vi "Data_get_joe.vi"() -> ()   [LabVIEW 2011]
uses:
  <vilib>/Analysis/2dsp.llb/Real FFT.vi
  <vilib>/Analysis/NI_AALPro.lvlib
panel:
  out "f cur. (GHz)":i32
  in  "TDS VISA Port":refnum<visa-resource-name>="GPIB0::1::INSTR"
  in  "Chirp up to (GHz)":dbl
  in  "PauseB":bool caption="Pause"
  in  "Substr":bool
  out "tdsavges#":i32 caption="tds averaged:"
  in  "Auto":bool caption="Autosave"
  in  "FFT every#":u32=1 min=1 max=1000 step=1
  in  "#steps":u32=1 min=1 step=1
  in  "f step (MHz)":dbl=0.0003 min=0.00025 max=67.0 step=1e-06 format="%#.12f"
  in  "time/point":T1(ring)
  in  "time/div":T2(ring)
  out "Current sweep":u32=1 min=1 max=1000 step=1
  in  "Ext":string="ccd"
  in  "Name":string="trace"
  in  "Folder":path
  in  "#Sweeps":u32=1 min=1 max=1000 step=1
  in  "Ampl. (dBm)":dbl min=-135.0 max=30.0 step=0.5 format="%#_8g"
  in  "f start (MHz)":dbl=0.0003 min=0.00025 max=67.0 step=1e-06 format="%#.12f"
  in  "Start":bool
  in  "Quit":bool
  in  "E8257D VISA Port":refnum<visa-resource-name>="GPIB0::1::INSTR"
  out "read time (ms)":u32
  out "#points":u32
  out "Busy":bool
  in  "Repetition rate (Hz)":ext=2.5
  in  "Chirp start (MHz)":ext=2.5
  in  "Filter up to (MHz)":ext=2.5
  in  "Amount of averagings":u32=10 min=1 step=1
  out "Data":dbl[](array[numeric])
  out "Frequency Domain Signal":cluster{ext[], dbl[]}(graph)
  out "FFT (Im)":dbl[](array[numeric])
  out "FFT (Re)":dbl[](array[numeric])
  out "Final array":ext[][](array[numeric])
  out "size(s)":i32
  out "Oscilloscope Data":dbl[](array[numeric])
  in  "Channel Number":u16=1
  out "Oscilloscope graph":dbl[](graph)
  in  "Stop":bool
  # "Oscilloscope TDS6124C"
  # "File Storage"
  # "PSG E8257D"
  # "Control"
  # "Spectrum data"
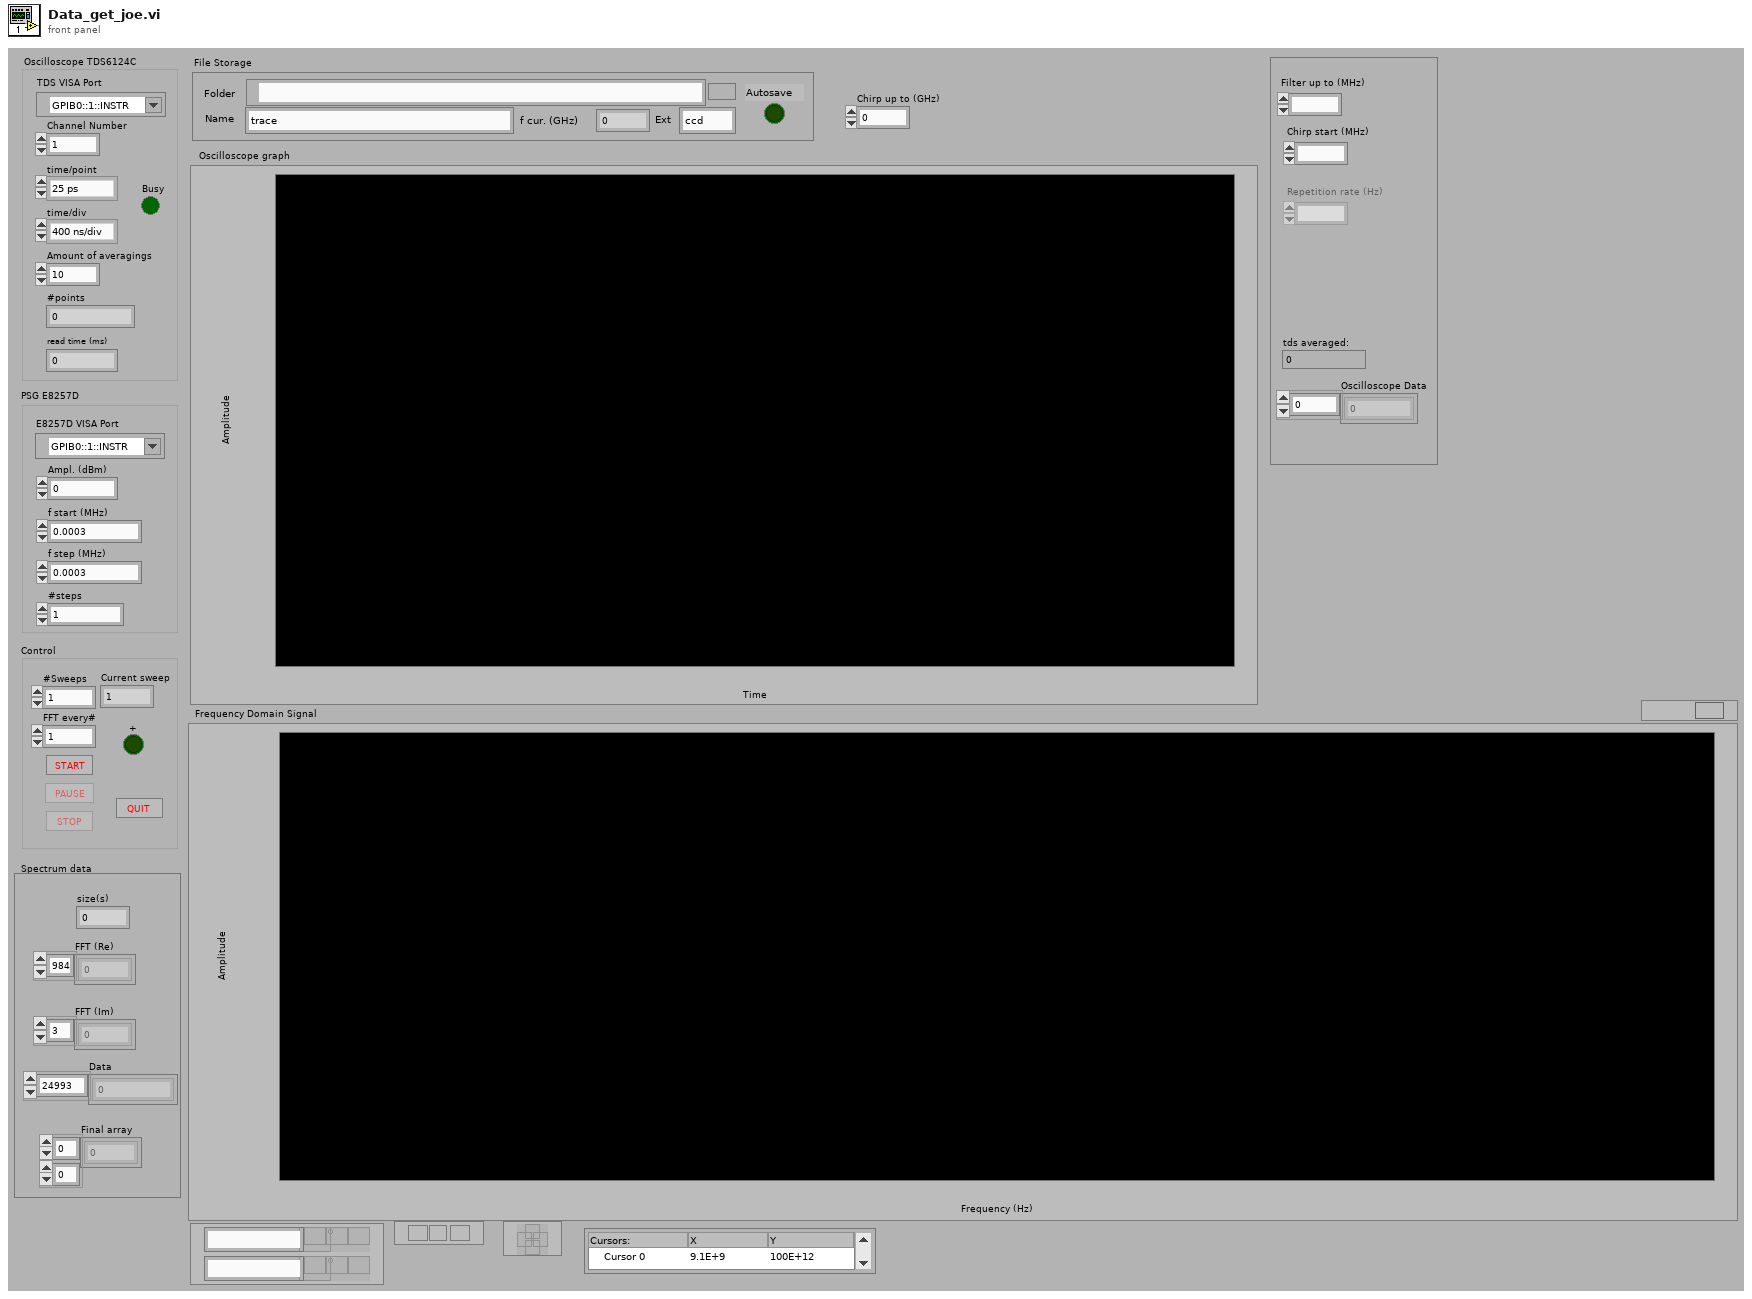
[diagram p1: front panel]
types:
  T1 = enum16{"25 ps", "50 ps", "100 ps", "200 ps", "400 ps", "800 ps", "2 ns"}
  T2 = enum16{"400 ns/div", "1 us/div", "2 us/div", "4 us/div", "10 us/div", "20 us/div"}
  T3 = enum8{"Enabled", "Disabled", "Disabled and Grayed Out"}
  T4 = enum16{"open", "replace", "create", "open or create", "replace or create", "replace or create with confirmation"}
  T5 = cluster{"Folder":path, "Name":string, "Ext":string}
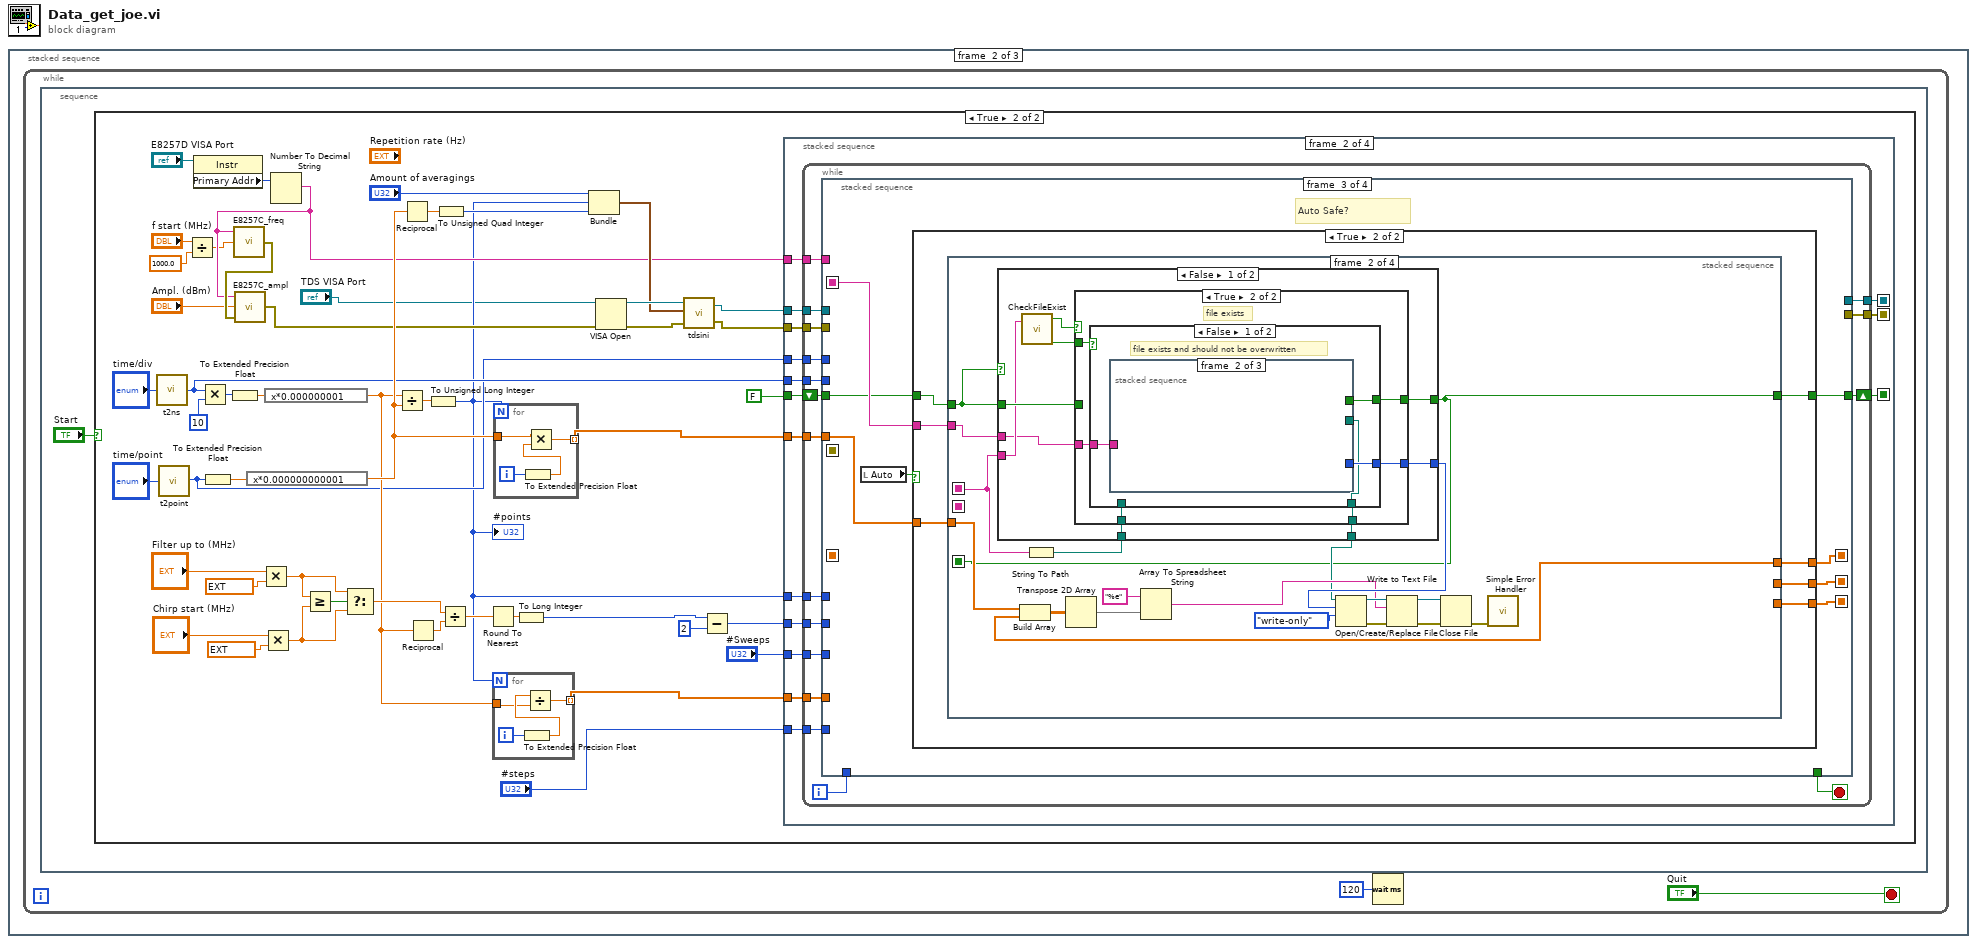
[diagram p0: block diagram]
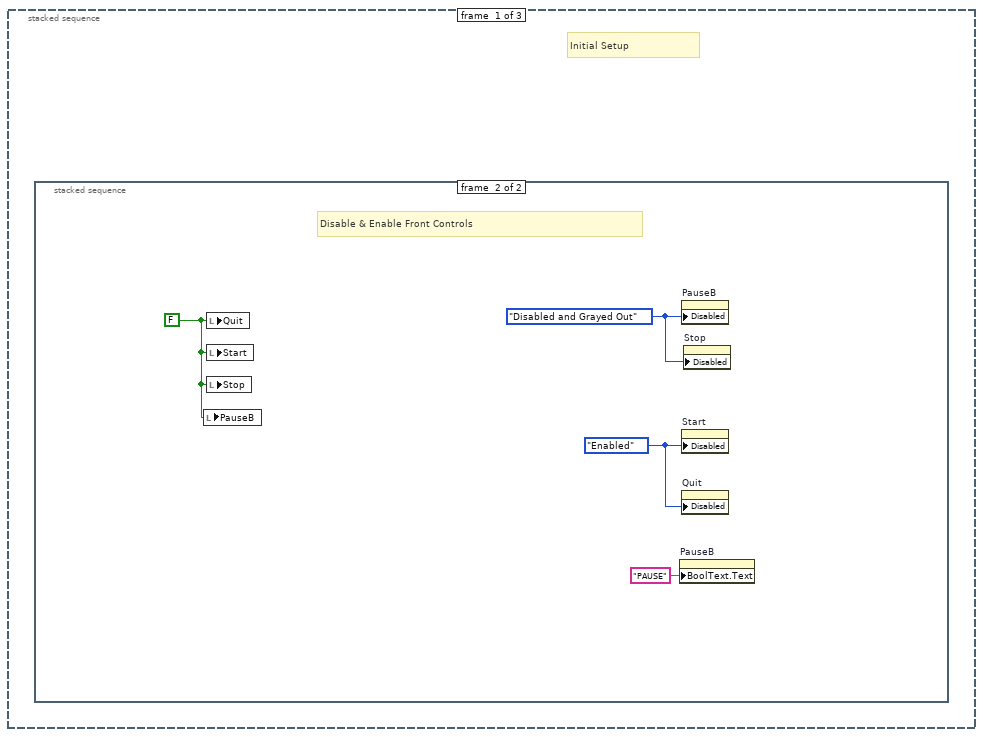
[diagram p2: hidden frame]
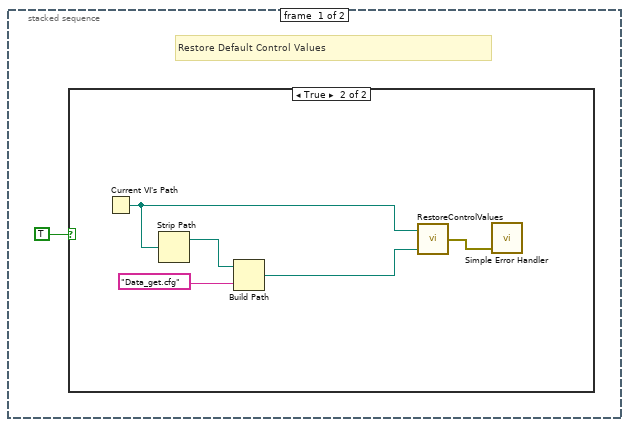
[diagram p3: hidden frame]
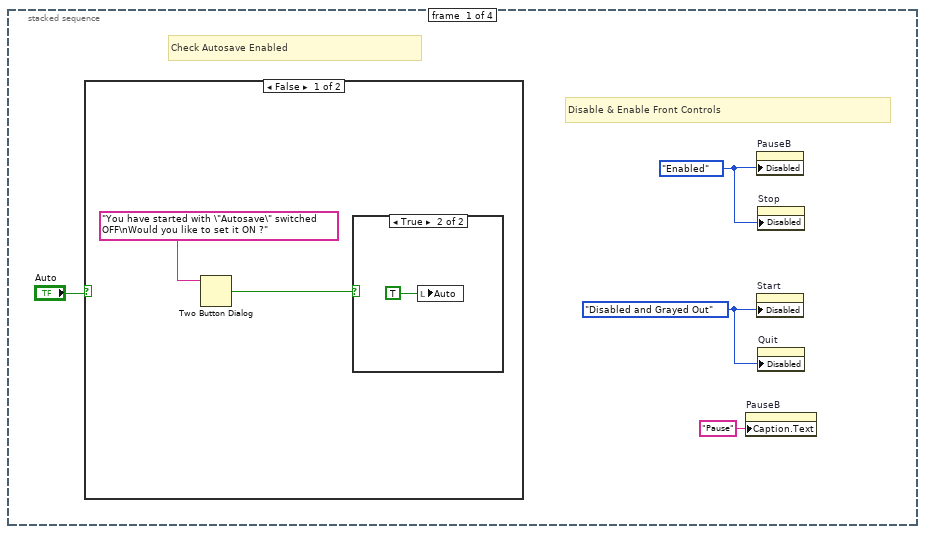
[diagram p6: hidden frame]
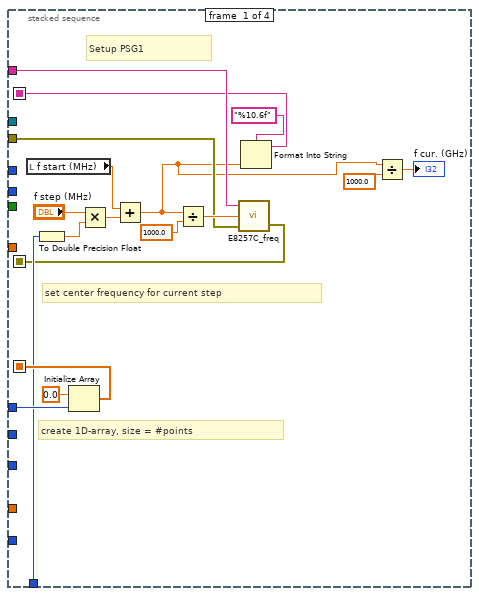
[diagram p9: hidden frame]
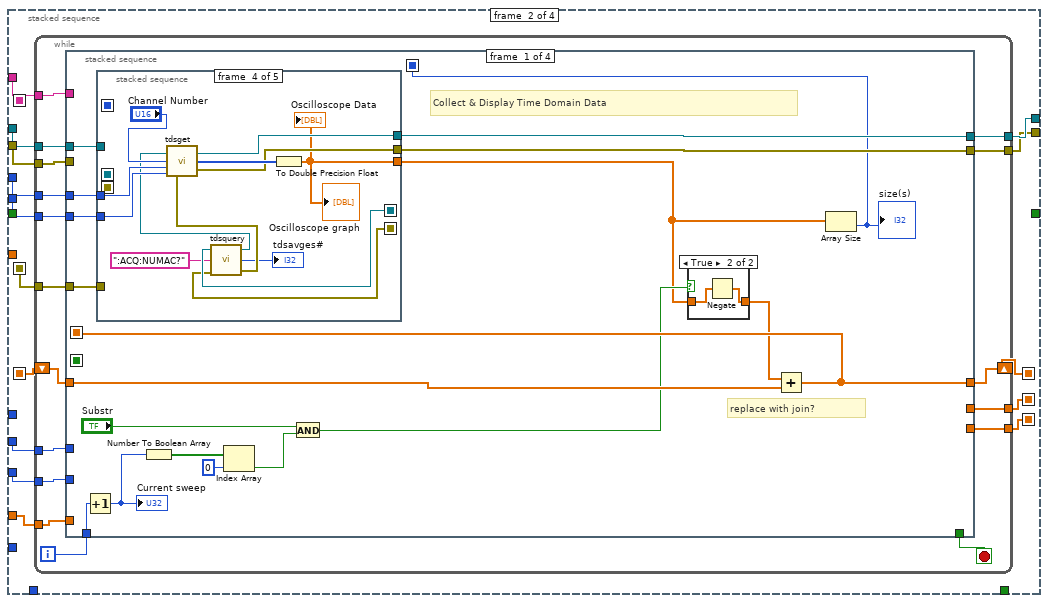
[diagram p10: hidden frame]
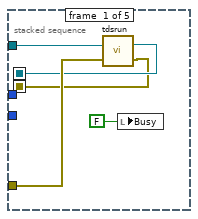
[diagram p12: hidden frame]
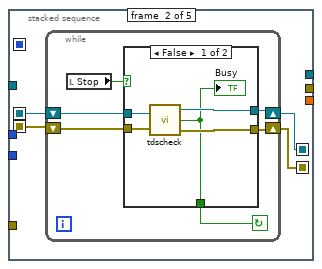
[diagram p13: hidden frame]
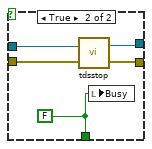
[diagram p14: hidden frame]
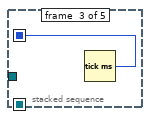
[diagram p15: hidden frame]
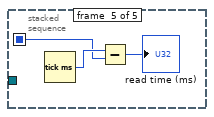
[diagram p16: hidden frame]
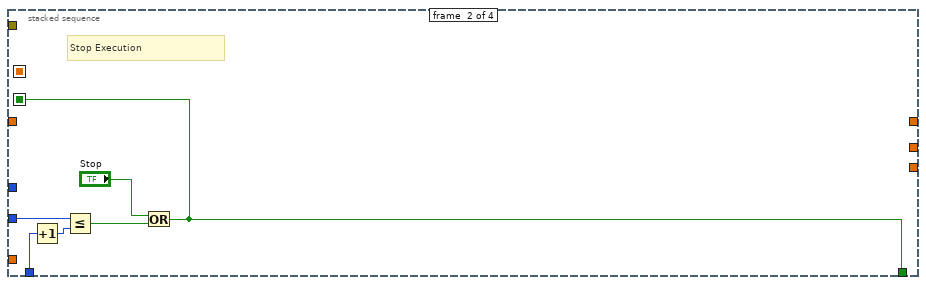
[diagram p17: hidden frame]
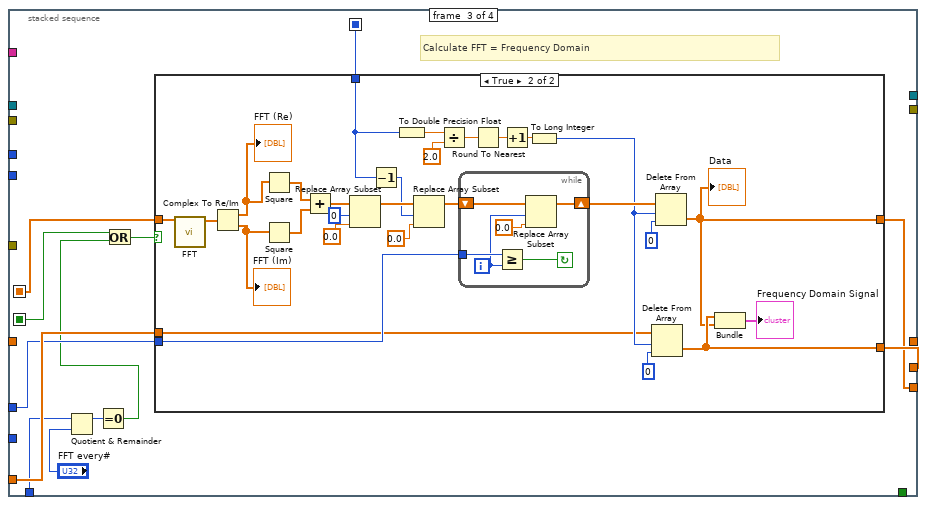
[diagram p18: hidden frame]
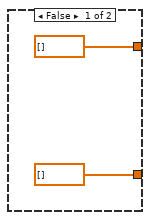
[diagram p19: hidden frame]
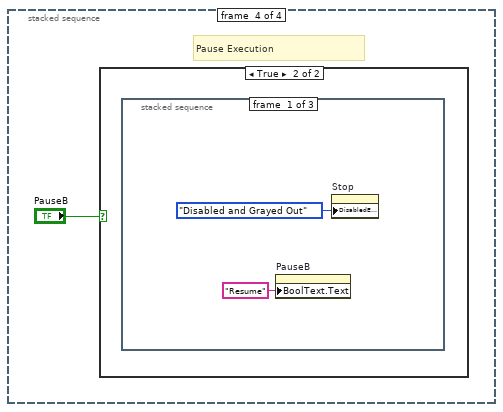
[diagram p20: hidden frame]
diagram:
  n1 = stacked-sequence {
    frame #0 {
      # "Initial Setup"
      n2 = stacked-sequence {
        frame #0 {
          # "Restore Default Control Values"
          n3 = case shown="True" TRUE {
            frame False {
            }
            frame True {
              n4 = Current VI's Path() -> (path=w2:path)
              n5 = Strip Path(path=w2) -> (stripped path=w3:path)  [unwired: 1 out]
              n6 = Build Path(base path=w3, name or relative path="Data_get.cfg") -> (appended path=w5:path)
              n7 = call "RestoreControlValues.vi"("file path"=w5, "vi path"=w2) -> ("error out"=w4:errorcluster)
              n8 = call <vilib>:"Simple Error Handler.vi"("error in (no error)"=w4) -> ()  [unwired: 4 in, 5 out]
            }
          }
        }
        frame #1 {
          w9 = T3."Disabled and Grayed Out" ("Disabled")
          w7 = T3."Enabled" ("Disabled")
          w10 = FALSE ("Quit")
          # "Disable & Enable Front Controls"
          n9 = local write "PauseB"(w10) -> ()
          n10 = local write "Quit"(w10) -> ()
          n11 = local write "Start"(w10) -> ()
          n12 = local write "Stop"(w10) -> ()
          n13 = property on="PauseB" class="Bool (strict)"("BoolText.Text"="PAUSE" ("Boolean Text.Text")) -> ()  [unwired: 2 in, 2 out]
          n14 = property on="PauseB" class="Bool (strict)"("Disabled"=w9) -> ()  [unwired: 2 in, 2 out]
          n15 = property on="Start" class="Bool (strict)"("Disabled"=w7) -> ()  [unwired: 2 in, 2 out]
          n16 = property on="Quit" class="Bool (strict)"("Disabled"=w7) -> ()  [unwired: 2 in, 2 out]
          n17 = property on="Stop" class="Bool (strict)"("Disabled"=w9) -> ()  [unwired: 2 in, 2 out]
        }
      }
    }
    frame #1 {
      n18 = while {
        stop <- "Quit" stop-if-true
        n19 = stacked-sequence {
          frame #0 {
            n20 = case shown="True" "Start" {
              frame False {
              }
              frame True {
                n21 = call "t2ns.vi"("t/div"="time/div") -> ("ns/div"=w25:u32)
                n22 = call "t2point.vi"("t/point"="time/point") -> ("ps/point"=w23:u32)
                n23 = Divide(x="f start (MHz)", y=1000.0) -> (x/y=w28:dbl)
                n24 = property class="Instr"(reference="E8257D VISA Port") -> ("Primary Addr"=w34:u16)  [unwired: 1 in, 2 out]
                n25 = Multiply(x=w25, y=u32 10) -> (x*y=w57:u32)
                n26 = To Extended Precision Float(1:w23) -> (0:w54:ext)
                n27 = To Extended Precision Float(1:w57) -> (0:w55:ext)
                n28 = expression code="x*0.000000000001"(w54) -> (w40:ext)
                n29 = Multiply(x="Filter up to (MHz)", y=ext 1000000.0) -> (x*y=w46:ext)
                n30 = Multiply(x="Chirp start (MHz)", y=ext 1000000.0) -> (x*y=w43:ext)
                n31 = expression code="x*0.000000001"(w55) -> (w36:ext)
                n32 = Number To Decimal String(number=w34) -> (decimal integer string=w31:string)  [unwired: 1 in]
                n33 = call "E8257C_freq.vi"("Frequency GHz"=w28, "GPIB address"=w31) -> ("error out"=w32:errorcluster)  [unwired: 1 in]
                n34 = call "E8257C_ampl.vi"("error in"=w32, "Amplitude dBm"="Ampl. (dBm)", "GPIB address"=w31) -> ("error out"=w30:errorcluster)
                n35 = Greater Or Equal?(x=w46, y=w43) -> (x >= y?=w53:bool)
                n36 = Select(t=w46, s=w53, f=w43) -> (s? t:f=w51:ext)
                n37 = Divide(x=w36, y=w40) -> (x/y=w56:ext)
                n38 = Reciprocal(x=w40) -> (1/x=w38:ext)
                n39 = Reciprocal(x=w36) -> (1/x=w52:ext)
                n40 = To Unsigned Long Integer(number=w56) -> (unsigned 32bit integer=w21:u32)
                "#points" <- w21
                n41 = To Unsigned Quad Integer(1:w38) -> (0:w39:u64)
                n42 = Divide(x=w51, y=w52) -> (x/y=w50:ext)
                n43 = Round To Nearest(number=w50) -> (nearest integer value=w49:ext)
                n44 = for {
                  N: w21 -> [_]
                  tunnel: w36 -> [w468]
                  tunnel: [w470] -> w37 mode=indexing
                  i -> [w471]
                  n45 = To Extended Precision Float(1:w471) -> (0:w469:ext)
                  n46 = Divide(x=w469, y=w468) -> (x/y=w470:ext)
                }
                n47 = for {
                  N: w21 -> [_]
                  tunnel: w40 -> [w473]
                  tunnel: [w472] -> w26 mode=indexing
                  i -> [w475]
                  n48 = To Extended Precision Float(1:w475) -> (0:w474:ext)
                  n49 = Multiply(x=w473, y=w474) -> (x*y=w472:ext)
                }
                n50 = To Long Integer(number=w49) -> (32bit integer=w18:i32)
                n51 = Bundle("Amount of averagings"="Amount of averagings", w21, w39) -> (w41:cluster{"Amount of averagings ":u32, u32, u64})  [unwired: 1 in]
                n52 = VISA Open(error in (no error)=w30, VISA resource name="TDS VISA Port") -> (VISA resource name=w59:refnum<visa-resource-name>, error out=w60:errorcluster)  [unwired: 3 in]
                n53 = call "tdsini.vi"("Error In (No Error)"=w60, "Acq_par"=w41, "VISA Port In"=w59) -> ("Error Out"=w61:errorcluster, "VISA Port Out"=w62:refnum<visa-resource-name>)
                n54 = Subtract(x=w18, y=2) -> (x-y=w16:i32)
                n55 = stacked-sequence {
                  seq-local: [_ w76 _ _] -> [_ _ w429 _]
                  seq-local: [_ w75 _ _] -> [_ _ w428 _]
                  seq-local: [_ w70 _ _] -> [_ _ _ w430]
                  tunnel: w62 -> [_ w84 _ _]
                  tunnel: w61 -> [_ w83 _ _]
                  tunnel: w23 -> [_ w82 _ _]
                  tunnel: w25 -> [_ w81 _ _]
                  tunnel: w16 -> [_ w80 _ _]
                  tunnel: w37 -> [_ w79 _ _]
                  tunnel: w31 -> [_ w78 w426 _]
                  tunnel: "#Sweeps" -> [_ w77 _ _]
                  tunnel: w26 -> [_ w72 _ _]
                  tunnel: w21 -> [_ w74 _ _]
                  tunnel: "#steps" -> [_ w73 _ _]
                  tunnel: FALSE -> [_ w71 _ _]
                  frame #0 {
                    w64 = T3."Enabled" ("Disabled")
                    w63 = T3."Disabled and Grayed Out" ("Disabled")
                    # "Check Autosave Enabled"
                    # "Disable & Enable Front Controls"
                    n56 = case shown="False" "Auto" {
                      frame False {
                        n57 = Two Button Dialog(message="You have started with \"Autosave\" switched OFF\nWould you like to set it ON ?") -> (T button?=w67:bool)  [unwired: 2 in]
                        n58 = case shown="True" w67 {
                          frame False {
                          }
                          frame True {
                            n59 = local write "Auto"(TRUE) -> ()
                          }
                        }
                      }
                      frame True {
                      }
                    }
                    n60 = property on="PauseB" class="Bool (strict)"("Caption.Text"="Pause") -> ()  [unwired: 2 in, 2 out]
                    n61 = property on="PauseB" class="Bool (strict)"("Disabled"=w64) -> ()  [unwired: 2 in, 2 out]
                    n62 = property on="Start" class="Bool (strict)"("Disabled"=w63) -> ()  [unwired: 2 in, 2 out]
                    n63 = property on="Stop" class="Bool (strict)"("Disabled"=w64) -> ()  [unwired: 2 in, 2 out]
                    n64 = property on="Quit" class="Bool (strict)"("Disabled"=w63) -> ()  [unwired: 2 in, 2 out]
                  }
                  frame #1 {
                    n65 = while {
                      tunnel: w84 -> [w101]
                      tunnel: w83 -> [w100]
                      tunnel: w82 -> [w99]
                      tunnel: w81 -> [w98]
                      tunnel: w80 -> [w97]
                      tunnel: w79 -> [w96]
                      tunnel: w78 -> [w95]
                      tunnel: w77 -> [w94]
                      tunnel: [w93] -> w76
                      tunnel: [w92] -> w75
                      tunnel: w74 -> [w91]
                      tunnel: w73 -> [w89]
                      tunnel: w72 -> [w87]
                      shift-right: [w85] -> w70
                      shift-left: w71 -> [w86]
                      i -> [w90]
                      stop <- w88 stop-if-true
                      n66 = stacked-sequence {
                        seq-local: [w118 _ _ _] -> [_ w124 _ _]
                        seq-local: [w107 _ _ _] -> [_ w123 _ _]
                        seq-local: [_ w122 _ _] -> [_ _ w282 _]
                        seq-local: [_ w121 _ _] -> [_ _ w281 _]
                        seq-local: [_ w120 _ _] -> [_ _ w280 _]
                        seq-local: [w105 _ _ _] -> [_ _ w279 _]
                        tunnel: w101 -> [_ w134 _ _]
                        tunnel: w100 -> [w108 w133 _ _]
                        tunnel: w99 -> [_ w132 _ _]
                        tunnel: w98 -> [_ w131 _ _]
                        tunnel: w97 -> [_ w130 _ _]
                        tunnel: w96 -> [_ w129 _ _]
                        tunnel: w95 -> [w109 w128 _ _]
                        tunnel: w94 -> [_ w127 _ _]
                        tunnel: [_ w126 _ _] -> w93
                        tunnel: [_ w125 _ _] -> w92
                        tunnel: w91 -> [w117 _ _ _]
                        tunnel: w90 -> [w112 _ _ w420]
                        tunnel: w89 -> [_ _ _ w419]
                        tunnel: [_ _ _ w418] -> w88
                        tunnel: w87 -> [_ _ w283 _]
                        tunnel: w86 -> [_ _ w277 _]
                        tunnel: [_ _ w276 _] -> w85
                        frame #0 {
                          # "Setup PSG1"
                          # "create 1D-array, size = #points"
                          # "set center frequency for current step"
                          n67 = local read "f start (MHz)"() -> (w110:dbl)
                          n68 = To Double Precision Float(number=w112) -> (double precision float=w113:dbl)
                          n69 = Initialize Array(0.0 ("element"), w117) -> (w118:dbl[])
                          n70 = Multiply(x="f step (MHz)", y=w113) -> (x*y=w111:dbl)
                          n71 = Add(x=w110, y=w111) -> (x+y=w103:dbl)
                          n72 = Divide(x=w103, y=1000.0) -> (x/y=w116:dbl)
                          n73 = call "E8257C_freq.vi"("error in"=w108, "Frequency GHz"=w116, "GPIB address"=w109) -> ("error out"=w107:errorcluster)
                          n74 = Format Into String(format string="%10.6f", w103) -> (resulting string=w105:string)  [unwired: 2 in, 1 out]
                          n75 = Divide(x=w103, y=1000.0) -> (x/y=→"f cur. (GHz)":dbl)
                        }
                        frame #1 {
                          n76 = while {
                            tunnel: [w148] -> w125
                            tunnel: [w149] -> w126
                            tunnel: w133 -> [w150]
                            tunnel: w134 -> [w151]
                            tunnel: w132 -> [w147]
                            tunnel: w131 -> [w146]
                            tunnel: w129 -> [w144]
                            tunnel: w130 -> [w145]
                            tunnel: w128 -> [w141]
                            tunnel: w127 -> [w140]
                            shift-right: [w138] -> w122
                            shift-left: w124 -> [w139]
                            tunnel: [w137] -> w121
                            tunnel: w123 -> [w136]
                            tunnel: [w135] -> w120
                            i -> [w143]
                            stop <- w142 stop-if-true
                            n77 = stacked-sequence {
                              seq-local: [w161 _ _ _] -> [_ _ w232 _]
                              seq-local: [w162 _ _ _] -> [_ _ w231 _]
                              seq-local: [_ w215 _ _] -> [_ _ w222 _]
                              tunnel: w151 -> [w169 _ _ _]
                              tunnel: w150 -> [_ _ _ _]
                              tunnel: [w168 _ _ _] -> w149
                              tunnel: [w167 _ _ _] -> w148
                              tunnel: w147 -> [w166 _ _ _]
                              tunnel: w146 -> [w165 _ _ _]
                              tunnel: w145 -> [_ _ w229 _]
                              tunnel: w144 -> [_ _ w230 _]
                              tunnel: w143 -> [w160 w220 w226 _]
                              tunnel: [_ w215 _ _] -> w142
                              tunnel: w141 -> [_ _ _ _]
                              tunnel: w140 -> [_ w217 _ _]
                              tunnel: w139 -> [w164 _ _ _]
                              tunnel: [w162 _ _ _] -> w138
                              tunnel: [_ _ w228 _] -> w137
                              tunnel: w136 -> [w163 _ _ _]
                              tunnel: [_ _ w227 _] -> w135
                              frame #0 {
                                # "replace with join?"
                                # "Collect & Display Time Domain Data"
                                n78 = Increment(x=w160) -> (x+1=w152:i32)
                                "Current sweep" <- w152
                                n79 = stacked-sequence {
                                seq-local: [w175 _ _ _ _] -> [_ w181 _ _ _]
                                seq-local: [w174 _ _ _ _] -> [_ w180 _ _ _]
                                seq-local: [_ w178 _ _ _] -> [_ _ _ w203 _]
                                seq-local: [_ w179 _ _ _] -> [_ _ _ w204 _]
                                seq-local: [_ _ w198 _ _] -> [_ _ _ _ w213]
                                tunnel: w169 -> [w176 _ _ _ _]
                                tunnel: w163 -> [w177 _ _ _ _]
                                tunnel: [_ _ _ w210 _] -> w168
                                tunnel: [_ _ _ w209 _] -> w167
                                tunnel: w166 -> [_ _ _ w207 _]
                                tunnel: w165 -> [_ _ _ w206 _]
                                tunnel: [_ _ _ w205 _] -> w155
                                frame #0 {
                                n80 = call "tdsrun.vi"("Error In (No Error)"=w177, "VISA Port In"=w176) -> ("Error Out"=w174:errorcluster, "VISA Port Out"=w175:refnum<visa-resource-name>)
                                n81 = local write "Busy"(FALSE ("Busy")) -> ()
                                }
                                frame #1 {
                                n82 = while {
                                shift-right: [w185] -> w179
                                shift-left: w181 -> [w186]
                                shift-right: [w184] -> w178
                                shift-left: w180 -> [w187]
                                stop <- w183 continue-if-true
                                n83 = local read "Stop"() -> (w182:bool)
                                n84 = case shown="False" w182 {
                                tunnel: w187 -> [w192 w196]
                                tunnel: w186 -> [w191 w197]
                                tunnel: [w190 w194] -> w185
                                tunnel: [w189 w195] -> w184
                                tunnel: [w188 w193] -> w183
                                frame False {
                                n85 = call "tdscheck.vi"("VISA Port In"=w191, "Error In (No Error)"=w192) -> ("VISA Port Out"=w190:refnum<visa-resource-name>, "busy"=w188:bool, "Error Out"=w189:errorcluster)
                                "Busy" <- w188
                                }
                                frame True {
                                w193 = FALSE ("busy")
                                n86 = call "tdsstop.vi"("Error In (No Error)"=w196, "VISA Port In"=w197) -> ("Error Out"=w195:errorcluster, "VISA Port Out"=w194:refnum<visa-resource-name>)
                                n87 = local write "Busy"(w193) -> ()
                                }
                                }
                                }
                                }
                                frame #2 {
                                n88 = Tick Count (ms)() -> (millisecond timer value=w198:u32)
                                }
                                frame #3 {
                                n89 = call "tdsquery.vi"("Error In (No Error)"=w203, "String to TDS"=":ACQ:NUMAC?", "VISA Port In"=w204) -> ("Error Out"=w200:errorcluster, "number"=→"tdsavges#":i32, "VISA Port Out"=w201:refnum<visa-resource-name>)
                                n90 = call "tdsget.vi"("VISA Port In"=w201, "Channel Number"="Channel Number", "ps/point"=w207, "ns/div"=w206, "Error In (No Error)"=w200) -> ("VISA Port Out"=w210:refnum<visa-resource-name>, "TDS Data"=w211:u16[], "Error Out"=w209:errorcluster)  [unwired: 8 in]
                                n91 = To Double Precision Float(number=w211) -> (double precision float=w205:dbl[])
                                "Oscilloscope graph" <- w205
                                "Oscilloscope Data" <- w205
                                }
                                frame #4 {
                                n92 = Tick Count (ms)() -> (millisecond timer value=w214:u32)
                                n93 = Subtract(x=w214, y=w213) -> (x-y=→"read time (ms)":u32)
                                }
                                }
                                n94 = Number To Boolean Array(number=w152) -> (Boolean array=w159:bool[])
                                n95 = Index Array(array=w159, index=0) -> (element=w157:bool)
                                n96 = And(x="Substr", y=w157) -> (x .and. y?=w156:bool)
                                n97 = case shown="True" w156 {
                                tunnel: w155 -> [w170 w172]
                                tunnel: [w170 w171] -> w154
                                frame False {
                                }
                                frame True {
                                n98 = Negate(x=w172) -> (-x=w171:dbl[])
                                }
                                }
                                n99 = Add(x=w154, y=w164) -> (x+y=w162:dbl[])
                                n100 = Array Size(array=w155) -> (size(s)=w161:i32)
                                "size(s)" <- w161
                              }
                              frame #1 {
                                # "Stop Execution"
                                n101 = Increment(x=w220) -> (x+1=w216:i32)
                                n102 = Less Or Equal?(x=w217, y=w216) -> (x <= y?=w219:bool)
                                n103 = Or(x="Stop", y=w219) -> (x .or. y?=w215:bool)
                              }
                              frame #2 {
                                # "Calculate FFT = Frequency Domain"
                                n104 = Quotient & Remainder(x=w226, y="FFT every#") -> (x-y*floor(x/y)=w224:u32)  [unwired: 1 out]
                                n105 = Equal To 0?(x=w224) -> (x = 0?=w221:bool)
                                n106 = Or(x=w222, y=w221) -> (x .or. y?=w223:bool)
                                n107 = case shown="True" w223 {
                                tunnel: w232 -> [_ w240]
                                tunnel: w231 -> [_ w239]
                                tunnel: w230 -> [_ w235]
                                tunnel: w229 -> [_ w238]
                                tunnel: [ext[] [] w237] -> w228
                                tunnel: [dbl[] [] w236] -> w227
                                frame False {
                                }
                                frame True {
                                n108 = call-poly <vilib>:"FFT.vi"("X"=w239) -> ("FFT {X}"=w262:cdb[])  [unwired: 9 in, 1 out]
                                n109 = Complex To Re/Im(x + iy=w262) -> (x=w261:dbl[], y=w260:dbl[])
                                "FFT (Re)" <- w261
                                "FFT (Im)" <- w260
                                n110 = Square(x=w261) -> (x^2=w259:dbl[])
                                n111 = Square(x=w260) -> (x^2=w258:dbl[])
                                n112 = Add(x=w259, y=w258) -> (x+y=w254:dbl[])
                                n113 = Replace Array Subset(array=w254, new element=0.0 ("new element/subarray"), index=0) -> (w253:dbl[])
                                n114 = Decrement(x=w240) -> (x-1=w252:i32)
                                n115 = To Double Precision Float(number=w240) -> (double precision float=w248:dbl)
                                n116 = Replace Array Subset(array=w253, new element=0.0 ("new element/subarray"), index=w252) -> (w250:dbl[])
                                n117 = Divide(x=w248, y=2.0) -> (x/y=w246:dbl)
                                n118 = while {
                                tunnel: w238 -> [w267]
                                shift-right: [w265] -> w249
                                shift-left: w250 -> [w266]
                                i -> [w264]
                                stop <- w268 continue-if-true
                                n119 = Greater Or Equal?(x=w267, y=w264) -> (x >= y?=w268:bool)
                                n120 = Replace Array Subset(array=w266, new element=0.0 ("new element/subarray"), index=w264) -> (w265:dbl[])
                                }
                                n121 = Round To Nearest(number=w246) -> (nearest integer value=w245:dbl)
                                n122 = Increment(x=w245) -> (x+1=w244:dbl)
                                n123 = To Long Integer(number=w244) -> (32bit integer=w241:i32)
                                n124 = Delete From Array(array=w235, length=w241, index=0) -> (deleted portion=w237:ext[])  [unwired: 1 out]
                                n125 = Delete From Array(array=w249, length=w241, index=0) -> (deleted portion=w236:dbl[])  [unwired: 1 out]
                                "Data" <- w236
                                n126 = Bundle(w237, w236) -> (→"Frequency Domain Signal":cluster{ext[], dbl[]})  [unwired: 1 in]
                                }
                                }
                              }
                              frame #3 {
                                # "Pause Execution"
                                n127 = case shown="True" "PauseB" {
                                frame False {
                                }
                                frame True {
                                n128 = stacked-sequence {
                                frame #0 {
                                n129 = property on="PauseB" class="Bool (strict)"("BoolText.Text"="Resume" ("Caption.Text")) -> ()  [unwired: 2 in, 2 out]
                                n130 = property on="Stop" class="Bool (strict)"("DisabledEnum"=T3."Disabled and Grayed Out" ("Disabled")) -> ()  [unwired: 2 in, 2 out]
                                }
                                frame #1 {
                                n131 = while {
                                stop <- w273 continue-if-true
                                n132 = local read "PauseB"() -> (w273:bool)
                                n133 = Wait Until Next ms Multiple(millisecond multiple=u32 150) -> ()  [unwired: 1 out]
                                }
                                }
                                frame #2 {
                                n134 = property on="PauseB" class="Bool (strict)"("BoolText.Text"="Pause" ("Caption.Text")) -> ()  [unwired: 2 in, 2 out]
                                n135 = property on="Stop" class="Bool (strict)"("DisabledEnum"=T3."Enabled" ("Disabled")) -> ()  [unwired: 2 in, 2 out]
                                }
                                }
                                }
                                }
                              }
                            }
                          }
                        }
                        frame #2 {
                          # "Auto Safe?"
                          n136 = local read "Auto"() -> (w278:bool)
                          n137 = case shown="True" w278 {
                            tunnel: w283 -> [_ w291]
                            tunnel: w282 -> [_ w290]
                            tunnel: w281 -> [_ w289]
                            tunnel: w280 -> [_ w288]
                            tunnel: w279 -> [_ w287]
                            tunnel: w277 -> [_ w286]
                            tunnel: [FALSE w285] -> w276
                            frame False {
                            }
                            frame True {
                              n138 = stacked-sequence {
                                seq-local: [w292 _ _ _] -> [_ w316 _ _]
                                seq-local: [_ _ w370 _] -> [_ _ _ w410]
                                seq-local: [_ w302 _ _] -> [_ _ _ w401]
                                tunnel: w291 -> [_ w318 _ _]
                                tunnel: w290 -> [_ w305 _ _]
                                tunnel: w289 -> [_ _ _ w413]
                                tunnel: w288 -> [_ _ _ w412]
                                tunnel: w287 -> [w295 w304 w372 _]
                                tunnel: w286 -> [_ w308 _ _]
                                tunnel: [_ w302 _ _] -> w285
                                frame #0 {
                                # "create complete filename incl. path as a string"
                                n139 = Path To String(path="Folder") -> (string=w300:string)
                                n140 = Concatenate Strings(w300, "\\\\" ("string"), "Name", "_", "td", w295, ".", "Ext") -> (w292:string)
                                }
                                frame #1 {
                                n141 = Build Array(w318, w305) -> (w320:ext[][])
                                n142 = String To Path(string=w316) -> (path=w307:path)
                                n143 = case shown="False" w308 {
                                tunnel: w316 -> [w322 _]
                                tunnel: [w327 w368] -> w302
                                tunnel: [w325 T4."replace or create" ("operation (0:open)")] -> w310
                                tunnel: w308 -> [w326 w368]
                                tunnel: w307 -> [w324 w367]
                                tunnel: [w323 w367] -> w306
                                tunnel: w304 -> [w321 _]
                                frame False {
                                n144 = call "CheckFileExist.vi"("Path"=w322) -> ("File Exists"=w329:bool, "Overwrite File"=w328:bool)  [unwired: 1 in, 1 out]
                                n145 = case "check file existance" shown="True" w329 {
                                tunnel: w328 -> [_ w338]
                                tunnel: [w332 w336] -> w327
                                tunnel: w326 -> [w332 _]
                                tunnel: [T4."create" ("operation (0:open)") w337] -> w325
                                tunnel: w324 -> [w330 w335]
                                tunnel: [w330 w334] -> w323
                                tunnel: w321 -> [_ w333]
                                frame False {
                                # "file doesn't exist"
                                }
                                frame True {
                                # "file exists"
                                n146 = case shown="False" w338 {
                                tunnel: [w341 T4."replace or create" ("operation (0:open)")] -> w337
                                tunnel: [w342 TRUE] -> w336
                                tunnel: w335 -> [_ w364]
                                tunnel: [w339 w364] -> w334
                                tunnel: w333 -> [w340 _]
                                frame False {
                                # "file exists and should not be overwritten"
                                n147 = stacked-sequence {
                                tunnel: [_ _ FALSE] -> w342
                                tunnel: [_ _ T4."create" ("operation (0:open)")] -> w341
                                tunnel: w340 -> [_ w351 _]
                                tunnel: [_ w356 _] -> w339
                                frame #0 {
                                # "enter new file name"
                                n148 = local read "Folder"() -> (w350:path)
                                n149 = local read "Name"() -> (w349:string)
                                n150 = local read "Ext"() -> (w348:string)
                                n151 = Bundle("Folder"=w350, "Name"=w349, "Ext"=w348) -> (w347:T5)  [unwired: 1 in]
                                n152 = call "ChangeFileName.vi"("input par"=w347) -> ("output par"=w346:T5)  [unwired: 1 out]
                                n153 = Unbundle(w346) -> ("Folder"=w345:path, "Name"=w344:string, "Ext"=w343:string)
                                n154 = local write "Folder"(w345) -> ()
                                n155 = local write "Name"(w344) -> ()
                                n156 = local write "Ext"(w343) -> ()
                                }
                                frame #1 {
                                # "create new path"
                                n157 = local read "Ext"() -> (w353:string)
                                n158 = local read "Folder"() -> (w358:path)
                                n159 = local read "Name"() -> (w357:string)
                                n160 = Path To String(path=w358) -> (string=w361:string)
                                n161 = Concatenate Strings(w361, "\\\\" ("string"), w357, "_", "td", w351, ".", w353) -> (w352:string)
                                n162 = String To Path(string=w352) -> (path=w356:path)
                                }
                                frame #2 {
                                }
                                }
                                }
                                frame True {
                                # "overwrite existing file"
                                }
                                }
                                }
                                }
                                }
                                frame True {
                                }
                                }
                                n163 = Transpose 2D Array(2D array=w320) -> (transposed array=w317:ext[][])
                                n164 = Array To Spreadsheet String(array=w317, 3:"%e") -> (spreadsheet string=w309:string)  [unwired: 1 in]
                                n165 = Open/Create/Replace File(file path (use dialog)=w306, operation (0:open)=w310, access (0:read/write)=enum16{"read/write", "read-only", "write-only"}."write-only") -> (refnum out=w312:refnum<file>, error out=w315:errorcluster)  [unwired: 3 in, 1 out]
                                n166 = Write to Text File(file (use dialog)=w312, text=w309, error in=w315) -> (refnum out=w313:refnum<file>, error out=w314:errorcluster)  [unwired: 1 in, 1 out]
                                n167 = Close File(refnum=w313, error in=w314) -> (error out=w303:errorcluster)  [unwired: 1 out]
                                n168 = call <vilib>:"Simple Error Handler.vi"("error in (no error)"=w303) -> ()  [unwired: 4 in, 5 out]
                                }
                                frame #2 {
                                n169 = local read "Folder"() -> (w374:path)
                                n170 = local read "Name"() -> (w373:string)
                                n171 = local read "Ext"() -> (w371:string)
                                n172 = Path To String(path=w374) -> (string=w380:string)
                                n173 = Concatenate Strings(w380, "\\\\" ("string"), w373, "_") -> (w375:string)
                                n174 = Concatenate Strings(w375, "sd", w372, ".", w371) -> (w370:string)
                                }
                                frame #3 {
                                n175 = Multiply(x="Chirp up to (GHz)", y=1000000000.0) -> (x*y=w382:dbl)
                                n176 = To Extended Precision Float(1:w382) -> (0:w381:ext)
                                n177 = To Extended Precision Float(1:w412) -> (0:w414:ext[])
                                n178 = Build Array(w413, w414) -> (w411:ext[][])
                                n179 = String To Path(string=w410) -> (path=w403:path)
                                n180 = case shown="True" w401 {
                                tunnel: [T4."replace or create with confirmation" ("operation (0:open)") T4."replace or create" ("operation (0:open)")] -> w402
                                frame False {
                                }
                                frame True {
                                }
                                }
                                n181 = Transpose 2D Array(2D array=w411) -> (transposed array=w384:ext[][])
                                n182 = Index Array(array=w384, index (col)=0 ("disabled index (col)")) -> (element=w394:ext[])  [unwired: 1 in]
                                n183 = Index Array(array=w394, index=1) -> (element=w396:ext)
                                n184 = Index Array(array=w394, index=0) -> (element=w395:ext)
                                n185 = Subtract(x=w396, y=w395) -> (x-y=w391:ext)
                                n186 = Divide(x=w381, y=w391) -> (x/y=w388:ext)
                                n187 = Round To Nearest(number=w388) -> (nearest integer value=w390:ext)
                                n188 = To Long Integer(number=w390) -> (32bit integer=w389:i32)
                                n189 = Increment(x=w389) -> (x+1=w385:i32)
                                n190 = Array Subset(array=w384, index (row)=0 ("index"), length (row)=w385, index (col)=0 ("index"), length (col)=w385) -> (w383:ext[][])
                                "Final array" <- w383
                                n191 = Array To Spreadsheet String(array=w383, 3:"%e") -> (spreadsheet string=w404:string)  [unwired: 1 in]
                                n192 = Open/Create/Replace File(file path (use dialog)=w403, operation (0:open)=w402, access (0:read/write)=enum16{"read/write", "read-only", "write-only"}."write-only") -> (refnum out=w406:refnum<file>, error out=w409:errorcluster)  [unwired: 3 in, 1 out]
                                n193 = Write to Text File(file (use dialog)=w406, text=w404, error in=w409) -> (refnum out=w407:refnum<file>, error out=w408:errorcluster)  [unwired: 1 in, 1 out]
                                n194 = Close File(refnum=w407, error in=w408) -> (error out=w400:errorcluster)  [unwired: 1 out]
                                n195 = call <vilib>:"Simple Error Handler.vi"("error in (no error)"=w400) -> ()  [unwired: 4 in, 5 out]
                                }
                              }
                            }
                          }
                        }
                        frame #3 {
                          n196 = Increment(x=w420) -> (x+1=w422:i32)
                          n197 = Less Or Equal?(x=w419, y=w422) -> (x <= y?=w423:bool)
                          n198 = local read "Stop"() -> (w421:bool)
                          n199 = Or(x=w421, y=w423) -> (x .or. y?=w418:bool)
                        }
                      }
                    }
                  }
                  frame #2 {
                    w425 = T3."Disabled and Grayed Out" ("Disabled")
                    w424 = T3."Enabled" ("Disabled")
                    n200 = call "E8257C_local.vi"("GPIB address"=w426) -> ("error out"=w427:errorcluster)  [unwired: 1 in]
                    n201 = call <vilib>:"Simple Error Handler.vi"("error in (no error)"=w427) -> ()  [unwired: 4 in, 5 out]
                    n202 = property on="Quit" class="Bool (strict)"("Disabled"=w424) -> ()  [unwired: 2 in, 2 out]
                    n203 = property on="PauseB" class="Bool (strict)"("Disabled"=w425) -> ()  [unwired: 2 in, 2 out]
                    n204 = property on="Stop" class="Bool (strict)"("Disabled"=w425) -> ()  [unwired: 2 in, 2 out]
                    n205 = property on="Start" class="Bool (strict)"("Disabled"=w424) -> ()  [unwired: 2 in, 2 out]
                    n206 = VISA Close(VISA resource name=w429, error in (no error)=w428) -> ()  [unwired: 1 out]
                  }
                  frame #3 {
                    n207 = local read "Auto"() -> (w431:bool)
                    n208 = case shown="False" w431 {
                      tunnel: w430 -> [_ w434]
                      frame False {
                      }
                      frame True {
                        n209 = local read "time/point"() -> (w463:T1)
                        n210 = local read "time/div"() -> (w462:T2)
                        n211 = local read "Channel Number"() -> (w464:u16)
                        n212 = local read "Amount of averagings"() -> (w461:u32)
                        n213 = local read "#Sweeps"() -> (w460:u32)
                        n214 = local read "Filter up to (MHz)"() -> (w459:ext)
                        n215 = local read "Chirp start (MHz)"() -> (w458:ext)
                        n216 = local read "Ampl. (dBm)"() -> (w457:dbl)
                        n217 = local read "f start (MHz)"() -> (w454:dbl)
                        n218 = local read "f step (MHz)"() -> (w453:dbl)
                        n219 = local read "#steps"() -> (w452:u32)
                        n220 = call "t2point.vi"("t/point"=w463) -> ("ps/point"=w455:u32)
                        n221 = call "t2ns.vi"("t/div"=w462) -> ("ns/div"=w456:u32)
                        n222 = local read "Folder"() -> (w448:path)
                        n223 = local read "Name"() -> (w447:string)
                        n224 = local read "Ext"() -> (w444:string)
                        n225 = Path To String(path=w448) -> (string=w451:string)
                        n226 = Format Into String(format string="Channel: %d\\nps/point: %d\\nns/div: %d\\nAmount of averagings: %d\\n#Sweeps: %d\\nFilter up to (MHz): %f\\nChirp start (MHz): %f\\nAmpl. (dBm): %f\\nf start (MHz): %f\\nf step (MHz): %f\\n#steps: %d\\n", w464, w455, w456, w461, w460, w459, w458, w457, w454, w453, w452) -> (resulting string=w435:string)  [unwired: 2 in, 1 out]
                        n227 = case shown="True" w434 {
                          tunnel: [T4."replace or create with confirmation" ("operation (0:open)") T4."replace or create" ("operation (0:open)")] -> w433
                          frame False {
                          }
                          frame True {
                          }
                        }
                        n228 = Concatenate Strings(w451, "\\\\" ("string"), w447, "_", "par", ".", w444) -> (w443:string)
                        n229 = String To Path(string=w443) -> (path=w437:path)
                        n230 = Open/Create/Replace File(file path (use dialog)=w437, operation (0:open)=w433, access (0:read/write)=enum16{"read/write", "read-only", "write-only"}."write-only") -> (refnum out=w439:refnum<file>, error out=w442:errorcluster)  [unwired: 3 in, 1 out]
                        n231 = Write to Text File(file (use dialog)=w439, text=w435, error in=w442) -> (refnum out=w440:refnum<file>, error out=w441:errorcluster)  [unwired: 1 in, 1 out]
                        n232 = Close File(refnum=w440, error in=w441) -> (error out=w438:errorcluster)  [unwired: 1 out]
                        n233 = call <vilib>:"Simple Error Handler.vi"("error in (no error)"=w438) -> ()  [unwired: 4 in, 5 out]
                      }
                    }
                    n234 = local write "Stop"(FALSE ("Stop")) -> ()
                  }
                }
              }
            }
          }
        }
        n235 = Wait (ms)(milliseconds to wait=u32 120) -> ()  [unwired: 1 out]
      }
    }
    frame #2 {
      n236 = Current VI's Path() -> (path=w476:path)
      n237 = Strip Path(path=w476) -> (stripped path=w477:path)  [unwired: 1 out]
      n238 = Build Path(base path=w477, name or relative path="Data_get.cfg") -> (appended path=w479:path)
      n239 = call "SaveControlValues.vi"("file path"=w479, "vi path"=w476) -> ("error out"=w478:errorcluster)
      n240 = call <vilib>:"Simple Error Handler.vi"("error in (no error)"=w478) -> ()  [unwired: 4 in, 5 out]
    }
  }
